vi "stability read_ONE_channel_specify_range_VISA.vi"(5 "postDAQ  wait ms":u32=12, 7 "preDAQ  wait ms":u32=25) -> (0 "error out":T1, 2 "data":dbl[](array[numeric]))   [LabVIEW 2024]
uses:
  <instrlib>/Keithley 6517/Keithley 6517.lvlib
panel:
  out "dt-m":dbl
  out "dt-s":dbl
  out "out":string
  out "log-error":errorcluster
  in  "stop":bool
  out "spreadsheet string":string
  out "meter-visa":refnum<visa-resource-name>
  out "Current Time:":string
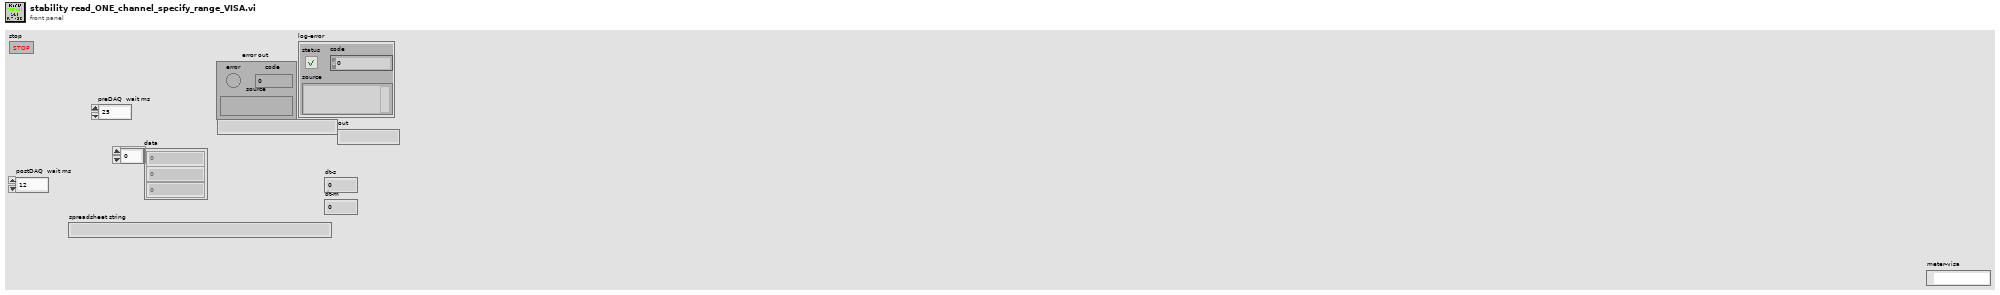
[diagram p1: front panel]
types:
  T1 = cluster{"error":bool, "code":i32, "source":string}
  T2 = enum16{"open", "replace", "create", "open or create", "replace or create", "replace or create with confirmation"}
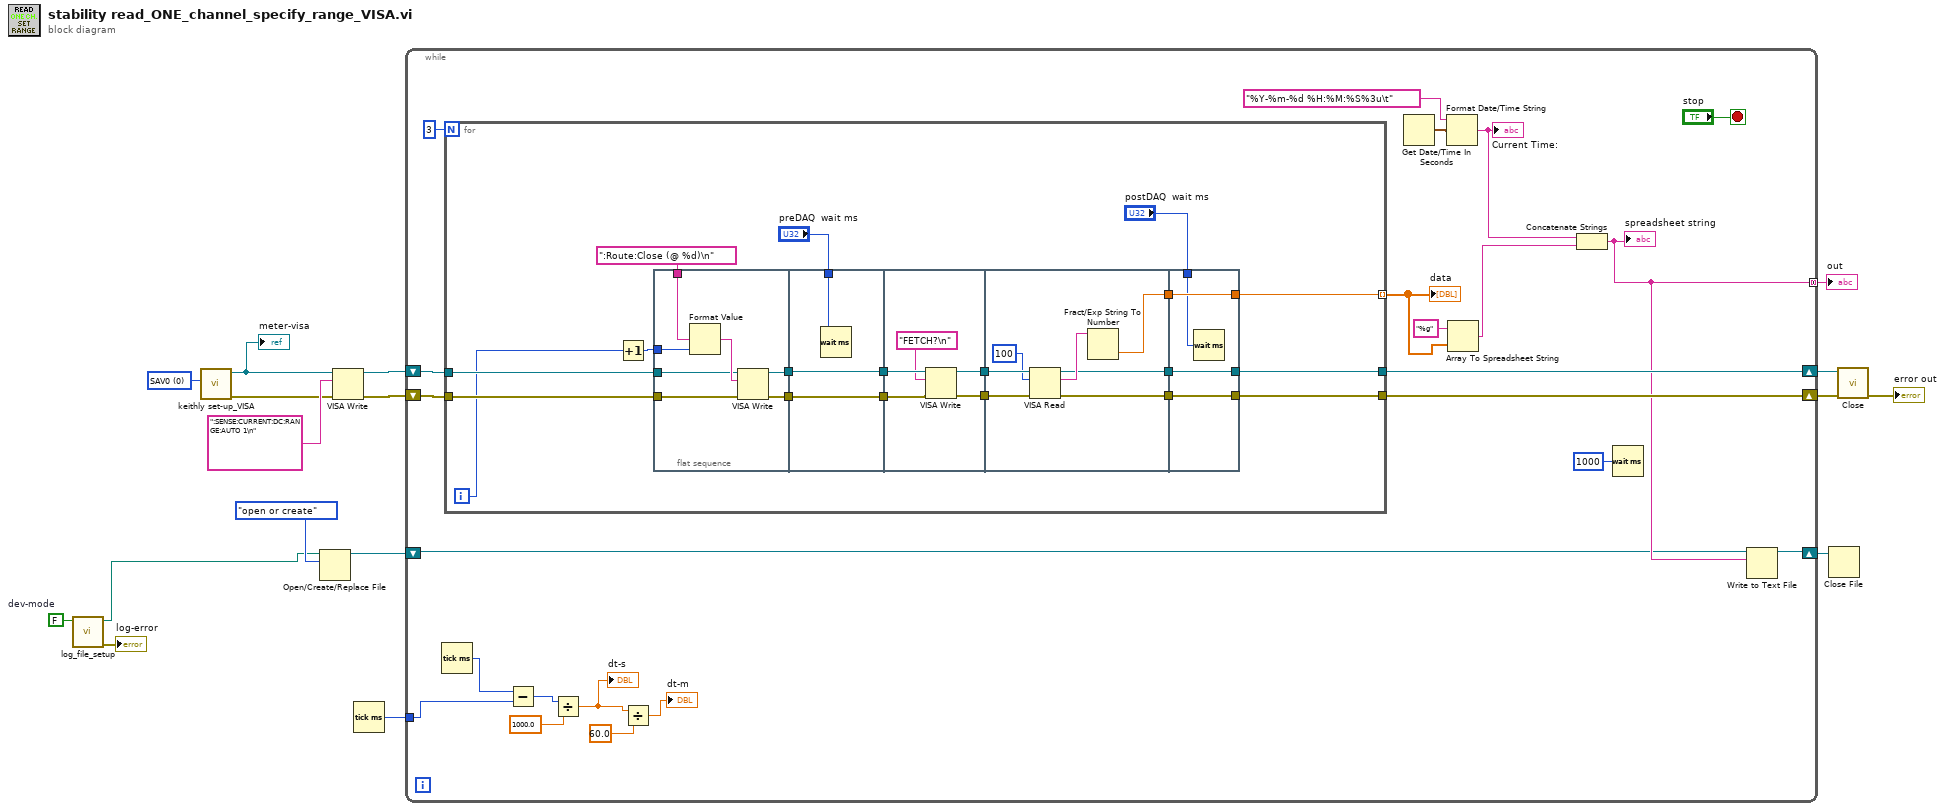
[diagram p0: block diagram]
diagram:
  w6 = FALSE  # dev-mode
  w14 = i16 0 items=["SAV0", "SAV1", "SAV2", "SAV3", "SAV4", "SAV5", "SAV6", "SAV7", "SAV8", "SAV9", "RST", "Preset"] ("ConfigOpt")
  n1 = call "log_file_setup.vi"("dev-mode"=w6) -> ("error out"=→"log-error":errorcluster, "appended path"=w7:path)  [unwired: 8 in, 1 out]
  n2 = call "keithly set-up_VISA.vi"("ConfigOpt"=w14) -> ("error out"=w12:errorcluster, "meter-VISA"=w13:refnum<visa-resource-name>)  [unwired: 9 in]
  "meter-visa" <- w13
  n3 = Open/Create/Replace File(file path (use dialog)=w7, operation (0:open)=T2."open or create") -> (refnum out=w4:refnum<file>)  [unwired: 4 in, 2 out]
  n4 = VISA Write(VISA resource name=w13, write buffer=":SENSE:CURRENT:DC:RANGE:AUTO 1\n", error in (no error)=w12) -> (VISA resource name out=w17:refnum<visa-resource-name>, error out=w15:errorcluster)  [unwired: 1 out]
  n5 = Tick Count (ms)() -> (millisecond timer value=w1:u32)
  n6 = while {
    shift-right: [w34] -> w9
    shift-left: w17 -> [w40]
    shift-right: [w35] -> w10
    shift-left: w15 -> [w39]
    tunnel: [w26] -> w2 mode=concatenating
    shift-right: [w27] -> w3
    shift-left: w4 -> [w25]
    tunnel: w1 -> [w23]
    stop <- "stop" stop-if-true
    n7 = Tick Count (ms)() -> (millisecond timer value=w24:u32)
    n8 = for {
      N: 3 -> [_]
      tunnel: [w50] -> w32 mode=indexing
      tunnel: w40 -> [w45]
      tunnel: w39 -> [w44]
      tunnel: [w42] -> w35
      tunnel: [w41] -> w34
      i -> [w43]
      n9 = Increment(x=w43) -> (x+1=w49:i32)
      n10 = flat-sequence {
        tunnel: [w66] -> w59
        tunnel: [w65] -> w58
        tunnel: w44 -> [w60]
        tunnel: ":Route:Close (@ %d)\n" -> [w61]
        tunnel: w45 -> [w63]
        tunnel: w49 -> [w62]
        tunnel: w59 -> [w69]
        tunnel: [w69] -> w57
        tunnel: "preDAQ  wait ms" -> [w68]
        tunnel: w58 -> [w67]
        tunnel: [w67] -> w56
        tunnel: w57 -> [w74]
        tunnel: w56 -> [w73]
        tunnel: [w71] -> w55
        tunnel: [w70] -> w54
        tunnel: [w77] -> w53
        tunnel: w55 -> [w81]
        tunnel: w54 -> [w80]
        tunnel: [w76] -> w52
        tunnel: [w75] -> w51
        tunnel: [w85] -> w50
        tunnel: w53 -> [w85]
        tunnel: "postDAQ  wait ms" -> [w84]
        tunnel: [w83] -> w41
        tunnel: w52 -> [w83]
        tunnel: [w82] -> w42
        tunnel: w51 -> [w82]
        frame #0 {
          n11 = Format Value(format string=w61, value (0)=w62) -> (output string=w64:string)  [unwired: 1 in]
          n12 = VISA Write(VISA resource name=w63, write buffer=w64, error in (no error)=w60) -> (VISA resource name out=w65:refnum<visa-resource-name>, error out=w66:errorcluster)  [unwired: 1 out]
        }
        frame #1 {
          n13 = Wait (ms)(milliseconds to wait=w68) -> ()  [unwired: 1 out]
        }
        frame #2 {
          n14 = VISA Write(VISA resource name=w73, write buffer="FETCH?\n", error in (no error)=w74) -> (VISA resource name out=w71:refnum<visa-resource-name>, error out=w70:errorcluster)  [unwired: 1 out]
        }
        frame #3 {
          n15 = VISA Read(VISA resource name=w81, byte count=u32 100, error in (no error)=w80) -> (VISA resource name out=w76:refnum<visa-resource-name>, read buffer=w78:string, error out=w75:errorcluster)  [unwired: 1 out]
          n16 = Fract/Exp String To Number(string=w78) -> (number=w77:dbl)  [unwired: 3 in, 1 out]
        }
        frame #4 {
          n17 = Wait (ms)(milliseconds to wait=w84) -> ()  [unwired: 1 out]
        }
      }
    }
    "data" <- w32
    n18 = Subtract(x=w24, y=w23) -> (x-y=w22:u32)
    n19 = Divide(x=w22, y=1000.0) -> (x/y=w19:dbl)
    "dt-s" <- w19
    n20 = Divide(x=w19, y=60.0) -> (x/y=→"dt-m":dbl)
    n21 = Get Date/Time In Seconds() -> (seconds since 1Jan1904=w37:timestamp)
    n22 = Format Date/Time String(time format string (%c)="%Y-%m-%d %H:%M:%S%3u\t", seconds (now)=w37) -> (date/time string=w31:string)  [unwired: 1 in]
    "Current Time:" <- w31
    n23 = Array To Spreadsheet String(array=w32, 3:"%g" ("format string")) -> (spreadsheet string=w30:string)  [unwired: 1 in]
    n24 = Concatenate Strings(w31, w30) -> (w26:string)
    "spreadsheet string" <- w26
    n25 = Wait (ms)(milliseconds to wait=u32 1000) -> ()  [unwired: 1 out]
    n26 = Write to Text File(file (use dialog)=w25, text=w26) -> (refnum out=w27:refnum<file>)  [unwired: 2 in, 2 out]
  }
  "out" <- w2
  n27 = Close File(refnum=w3) -> ()  [unwired: 1 in, 2 out]
  n28 = call <instrlib>:"Close.vi"("error in (no error)"=w10, "VISA resource name"=w9) -> ("error out"=→"error out":errorcluster)  [unwired: 9 in]
